vi "M100DailyOutputAuto.vi"() -> ()   [LabVIEW 2012]
uses:
  <vilib>/addons/database/Connection.llb/DB Tools Open Connec (Path).vi
  <vilib>/addons/database/Connection.llb/Conn Execute.vi
  <vilib>/addons/database/Recordset.llb/Rec Fetch Recordset Data (R).vi
  <vilib>/addons/database/Recordset.llb/Rec Destroy - Connection.vi
  <vilib>/Utility/file.llb/Write To Spreadsheet File (string).vi
  <vilib>/addons/database/_DB Variant To Data/Database Variant To Data.xnode
  <vilib>/addons/database/NI_Database_API.lvlib
  <vilib>/Utility/SMTP/NI_SMTPEmail.lvlib
panel:
  out "error out":errorcluster
  out "Array 2":string[][](array[string])
  out "spreadsheet string":string
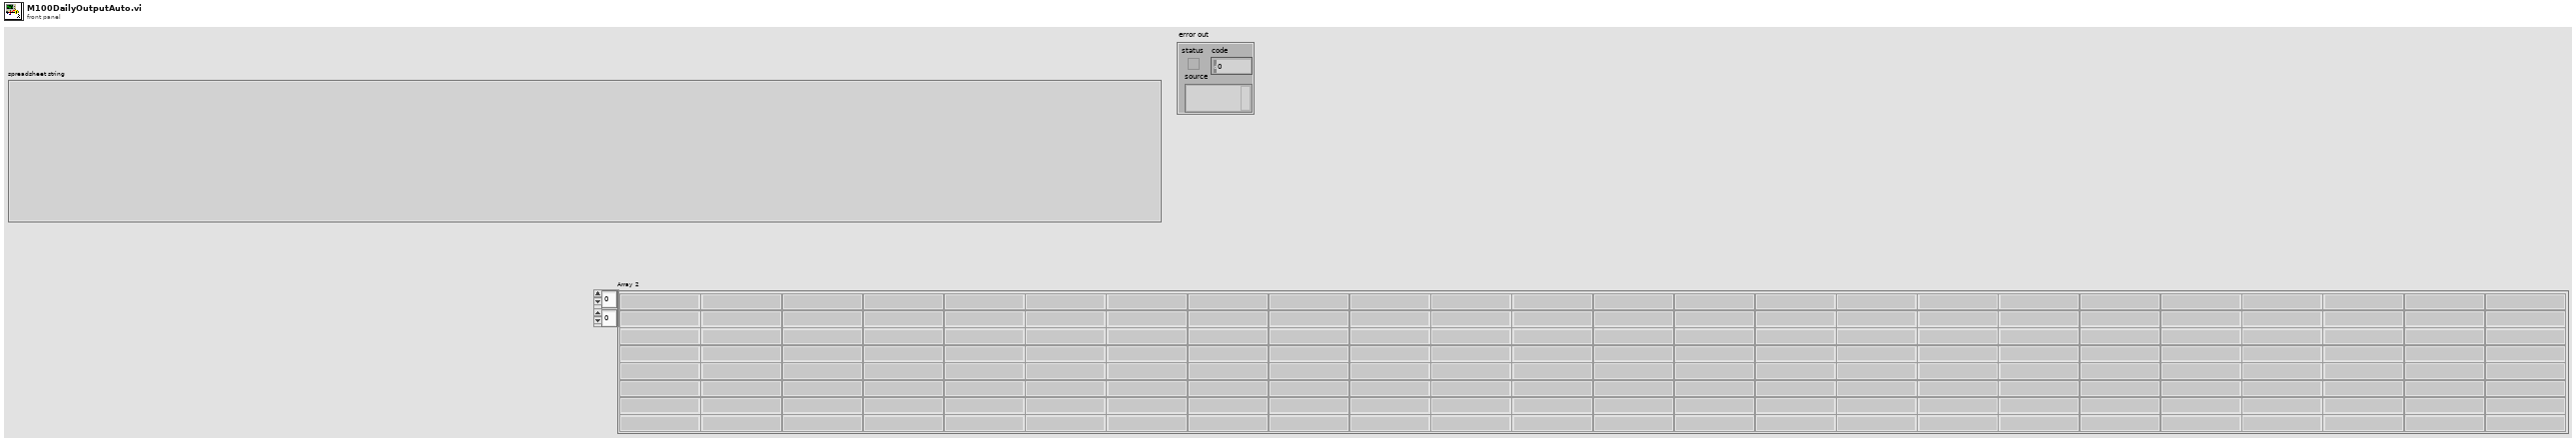
[diagram p1: front panel]
types:
  T1 = typedef "NI_Database_API.lvlib/Conn ObjectReference.ctl" = refnum<k1>
  T2 = typedef "NI_Database_API.lvlib/Rec ObjectReference.ctl" = refnum<k1>
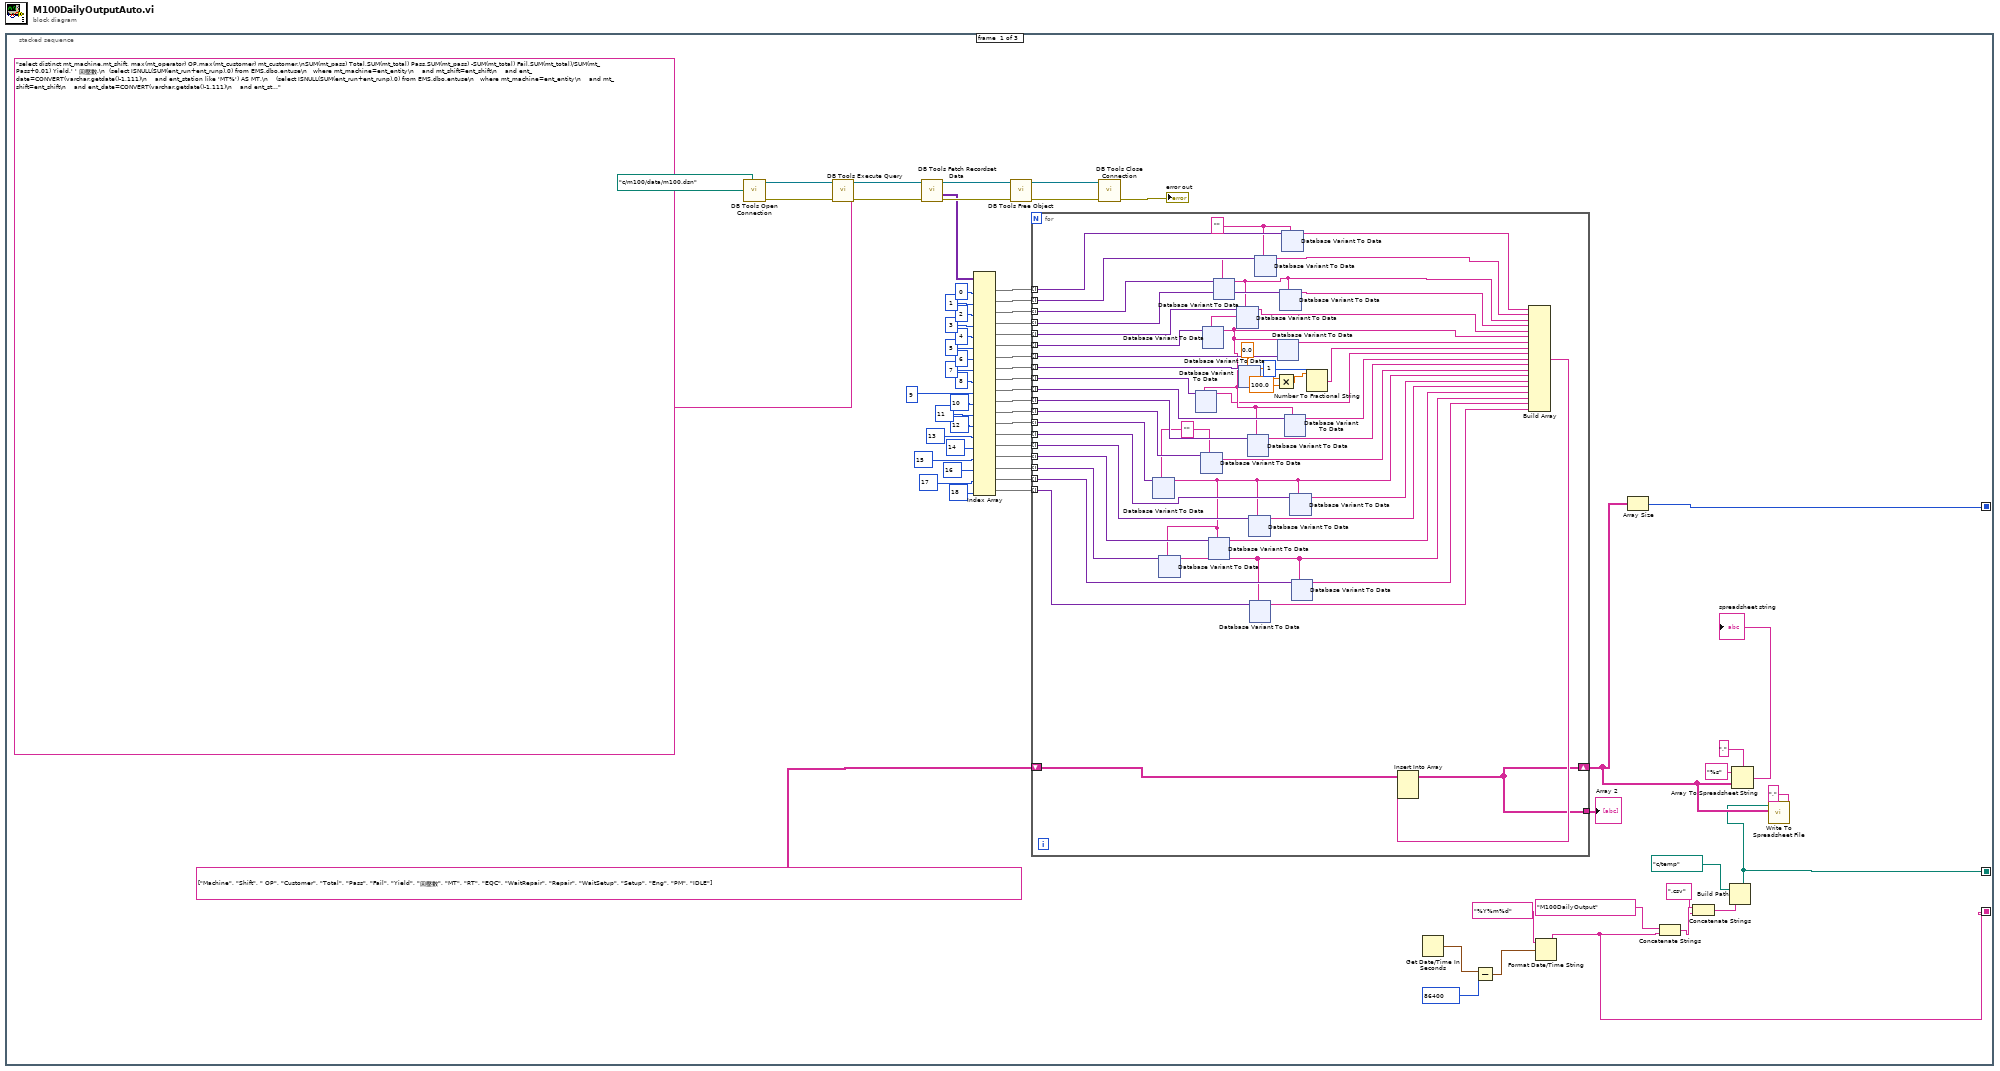
[diagram p0: block diagram]
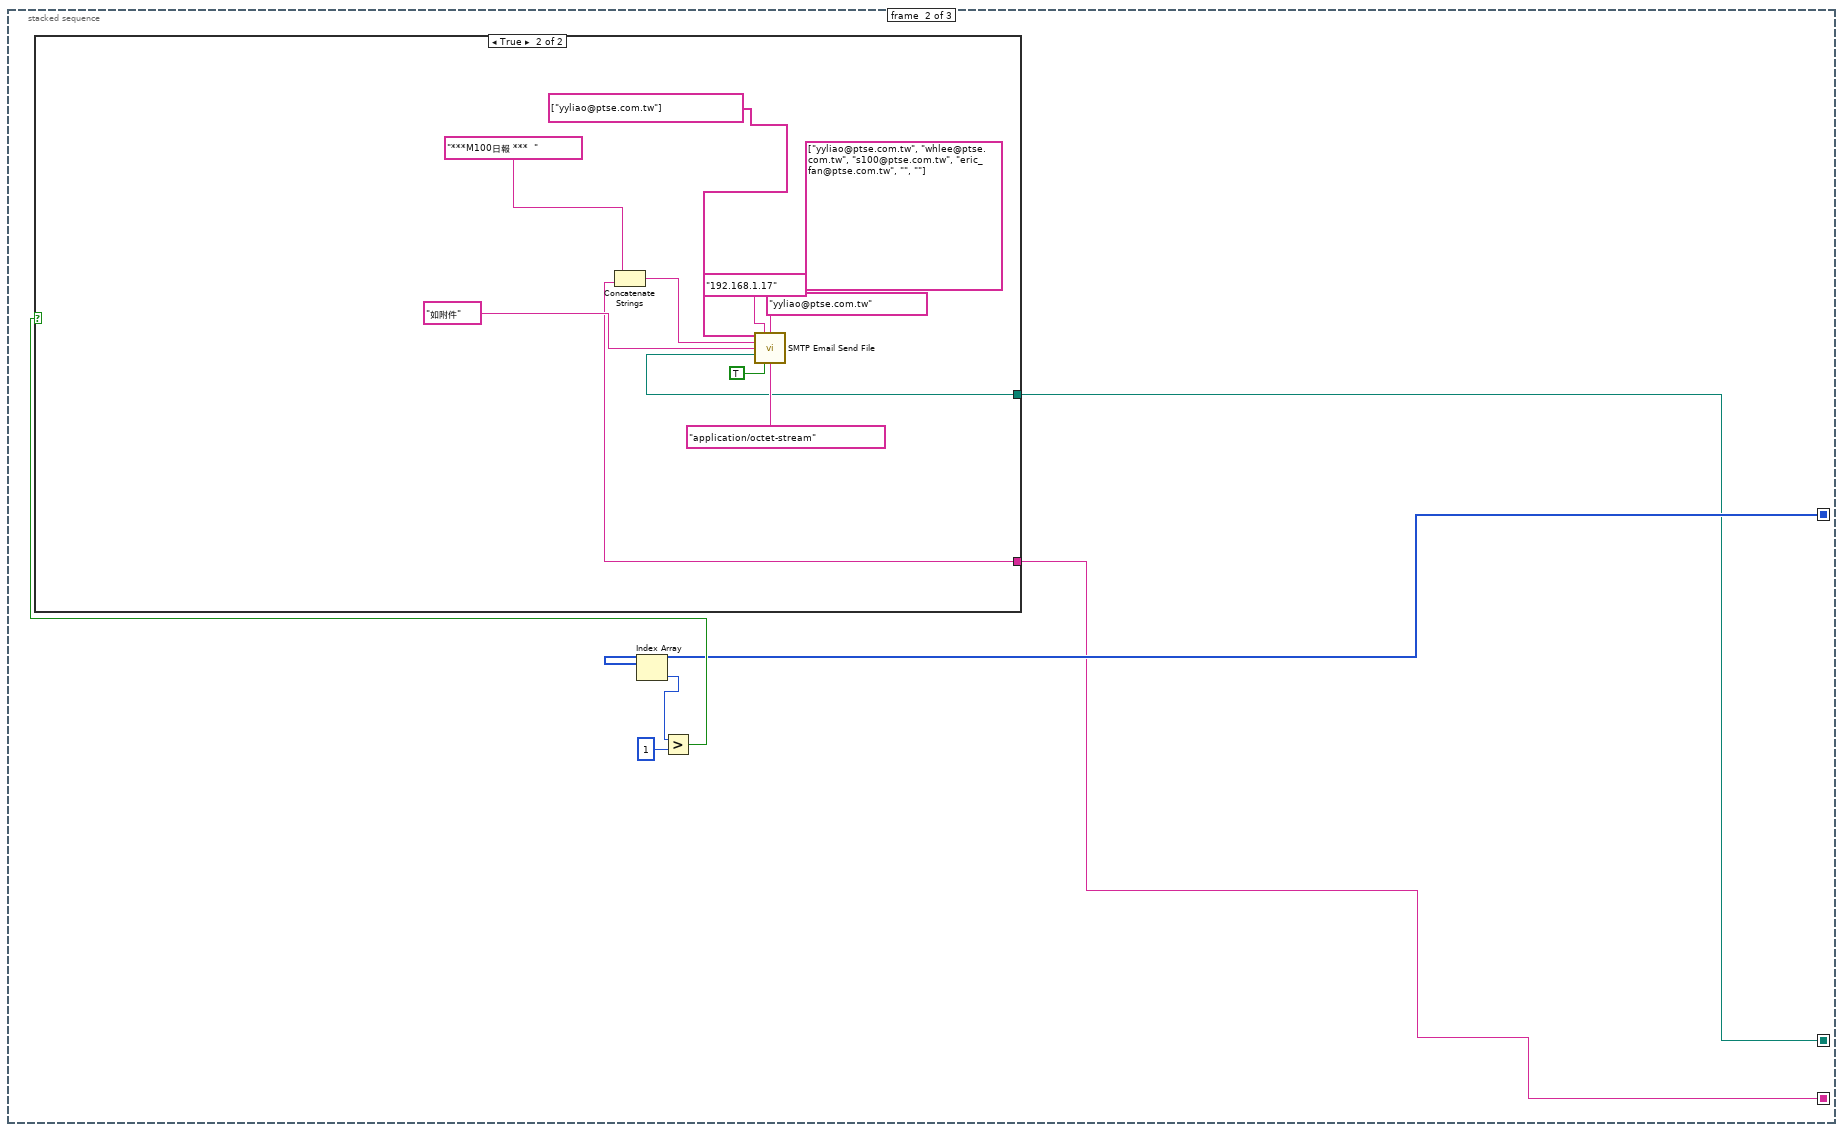
[diagram p2: hidden frame]
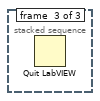
[diagram p4: hidden frame]
diagram:
  n1 = stacked-sequence {
    seq-local: [w37 _ _] -> [_ w728 _]
    seq-local: [w8 _ _] -> [_ w727 _]
    seq-local: [w4 _ _] -> [_ w726 _]
    frame #0 {
      n2 = call-poly <vilib>:"DB Tools Open Connection.vi"("connection information"=path "c:/m100/data/m100.dsn") -> ("error out"=w64:errorcluster, "connection reference"=w68:T1)  [unwired: 7 in]
      n3 = call-poly <vilib>:"DB Tools Execute Query.vi"("error in (no error)"=w64, "SQL query"="select distinct mt_machine,mt_shift, max(mt_operator) OP,max(mt_customer) mt_customer,\nSUM(mt_pass) Total,SUM(mt_total) Pass,SUM(mt_pass) -SUM(mt_total) Fail,SUM(mt_total)/SUM(mt_Pass+0.01) Yield,' ' 回壓數,\n  (select ISNULL(SUM(ent_run+ent_runp),0) from EMS.dbo.entuse\n   where mt_machine=ent_entity\n    and mt_shift=ent_shift\n    and ent_date=CONVERT(varchar,getdate()-1,111)\n    and ent_station like 'MT%') AS MT,\n    (select ISNULL(SUM(ent_run+ent_runp),0) from EMS.dbo.entuse\n   where mt_machine=ent_entity\n    and mt_shift=ent_shift\n    and ent_date=CONVERT(varchar,getdate()-1,111)\n    and ent_station like 'RT%') AS RT,\n    (select ISNULL(SUM(ent_run+ent_runp),0) from EMS.dbo.entuse\n   where mt_machine=ent_entity\n    and mt_shift=ent_shift\n    and ent_date=CONVERT(varchar,getdate()-1,111)\n    and ent_station like 'EQ%') AS EQC,\n    (select ISNULL(SUM(ent_wait_repair),0) from EMS.dbo.entuse\n   where mt_machine=ent_entity\n    and mt_shift=ent_shift\n    and ent_date=CONVERT(varchar,getdate()-1,111)) as WaitRepair,\n     (select ISNULL(SUM(ent_repair),0) from EMS.dbo.entuse\n   where mt_machine=ent_entity\n    and mt_shift=ent_shift\n    and ent_date=CONVERT(varchar,getdate()-1,111)) as Repair,\n    (select ISNULL(SUM(ent_wait_setup),0) from EMS.dbo.entuse\n   where mt_machine=ent_entity\n    and mt_shift=ent_shift\n    and ent_date=CONVERT(varchar,getdate()-1,111)) as WaitSetup,\n     (select ISNULL(SUM(ent_setup),0) from EMS.dbo.entuse\n   where mt_machine=ent_entity\n    and mt_shift=ent_shift\n    and ent_date=CONVERT(varchar,getdate()-1,111)) as Setup,\n    (select ISNULL(SUM(ent_eng),0) from EMS.dbo.entuse\n   where mt_machine=ent_entity\n    and mt_shift=ent_shift\n    and ent_date=CONVERT(varchar,getdate()-1,111)) as Eng,\n     (select ISNULL(SUM(ent_pm),0) from EMS.dbo.entuse\n   where mt_machine=ent_entity\n    and mt_shift=ent_shift\n    and ent_date=CONVERT(varchar,getdate()-1,111)) as PM,\n    (select ISNULL(SUM(ent_idle),0) from EMS.dbo.entuse\n   where mt_machine=ent_entity\n    and mt_shift=ent_shift\n    and ent_date=CONVERT(varchar,getdate()-1,111)) as IDLE\n  from m100.dbo.mt_data\n  where CONVERT(varchar,mt_end,111)=CONVERT(varchar,getdate()-1,111)\n    and mt_machine like 'QAMT%'\n  group by mt_machine,mt_shift\n  order by mt_machine,mt_shift desc", "connection reference"=w68) -> ("error out"=w63:errorcluster, "recordset reference"=w67:T2)  [unwired: 5 in]
      n4 = call-poly <vilib>:"DB Tools Fetch Recordset Data.vi"("error in (no error)"=w63, "recordset reference"=w67) -> ("error out"=w62:errorcluster, "recordset data"=w31:variant[][], "recordset reference out"=w66:T2)  [unwired: 3 in]
      n5 = Index Array(array=w31, index (col) #1=0 ("disabled index (col)"), index (col) #2=1 ("index (col)"), index (col) #3=2 ("index (col)"), index (col) #4=3 ("index (col)"), index (col) #5=4 ("index (col)"), index (col) #6=5 ("index (col)"), index (col) #7=6 ("index (col)"), index (col) #8=7 ("index (col)"), index (col) #9=8 ("index (col)"), index (col) #10=9 ("index (col)"), index (col) #11=10 ("index (col)"), index (col) #12=11 ("index (col)"), index (col) #13=12 ("index (col)"), index (col) #14=13 ("index (col)"), index (col) #15=14 ("index (col)"), index (col) #16=15 ("index (col)"), index (col) #17=16 ("index (col)"), index (col) #18=17 ("index (col)"), index (col) #19=18 ("index (col)")) -> (element #1=w48:variant[], element #2=w47:variant[], element #3=w46:variant[], element #4=w45:variant[], element #5=w44:variant[], element #6=w43:variant[], element #7=w42:variant[], element #8=w41:variant[], element #9=w40:variant[], element #10=w39:variant[], element #11=w38:variant[], element #12=w34:variant[], element #13=w33:variant[], element #14=w25:variant[], element #15=w24:variant[], element #16=w23:variant[], element #17=w22:variant[], element #18=w21:variant[], element #19=w1:variant[])  [unwired: 19 in]
      n6 = call-poly <vilib>:"DB Tools Free Object.vi"("error in (no error)"=w62, "recordset reference"=w66) -> ("error out"=w61:errorcluster, "connection reference"=w65:T1)  [unwired: 8 in]
      n7 = for {
        tunnel: w48 -> [w117] mode=indexing
        tunnel: w47 -> [w116] mode=indexing
        tunnel: w46 -> [w115] mode=indexing
        tunnel: w45 -> [w114] mode=indexing
        tunnel: w44 -> [w113] mode=indexing
        tunnel: w43 -> [w112] mode=indexing
        tunnel: w42 -> [w111] mode=indexing
        tunnel: w41 -> [w110] mode=indexing
        tunnel: w40 -> [w109] mode=indexing
        tunnel: w39 -> [w108] mode=indexing
        tunnel: w38 -> [w107] mode=indexing
        tunnel: [w104] -> w20
        shift-right: [w104] -> w16
        shift-left: string[][] [["Machine", "Shift", " OP", "Customer", "Total", "Pass", "Fail", "Yield", "回壓數", "MT", "RT", "EQC", "WaitRepair", "Repair", "WaitSetup", "Setup", "Eng", "PM", "IDLE"]] ("Array") -> [w103]
        tunnel: w34 -> [w102] mode=indexing
        tunnel: w33 -> [w101] mode=indexing
        tunnel: w25 -> [w88] mode=indexing
        tunnel: w24 -> [w87] mode=indexing
        tunnel: w23 -> [w86] mode=indexing
        tunnel: w22 -> [w85] mode=indexing
        tunnel: w21 -> [w84] mode=indexing
        tunnel: w1 -> [w78] mode=indexing
        w100 = ""
        w97 = ""
        n8 = xnode "Database Variant To Data"("database variant"=w101, "type"=w100) -> ("data"=w83:string)  [unwired: 1 in, 1 out]
        n9 = xnode "Database Variant To Data"("database variant"=w85, "type"=w83) -> ("data"=w77:string)  [unwired: 1 in, 1 out]
        n10 = xnode "Database Variant To Data"("database variant"=w102, "type"=w100) -> ("data"=w99:string)  [unwired: 1 in, 1 out]
        n11 = xnode "Database Variant To Data"("database variant"=w86, "type"=w83) -> ("data"=w80:string)  [unwired: 1 in, 1 out]
        n12 = xnode "Database Variant To Data"("database variant"=w115, "type"=w97) -> ("data"=w94:string)  [unwired: 1 in, 1 out]
        n13 = xnode "Database Variant To Data"("database variant"=w112, "type"=w94) -> ("data"=w93:string)  [unwired: 1 in, 1 out]
        n14 = xnode "Database Variant To Data"("database variant"=w109, "type"=w93) -> ("data"=w91:string)  [unwired: 1 in, 1 out]
        n15 = xnode "Database Variant To Data"("database variant"=w113, "type"=w94) -> ("data"=w95:string)  [unwired: 1 in, 1 out]
        n16 = xnode "Database Variant To Data"("database variant"=w110, "type"=0.0) -> ("data"=w74:dbl)  [unwired: 1 in, 1 out]
        n17 = xnode "Database Variant To Data"("database variant"=w107, "type"=w93) -> ("data"=w89:string)  [unwired: 1 in, 1 out]
        n18 = xnode "Database Variant To Data"("database variant"=w87, "type"=w83) -> ("data"=w81:string)  [unwired: 1 in, 1 out]
        n19 = xnode "Database Variant To Data"("database variant"=w78, "type"=w77) -> ("data"=w76:string)  [unwired: 1 in, 1 out]
        n20 = xnode "Database Variant To Data"("database variant"=w116, "type"=w97) -> ("data"=w98:string)  [unwired: 1 in, 1 out]
        n21 = Multiply(x=w74, y=100.0) -> (x*y=w72:dbl)
        n22 = xnode "Database Variant To Data"("database variant"=w111, "type"=w93) -> ("data"=w92:string)  [unwired: 1 in, 1 out]
        n23 = xnode "Database Variant To Data"("database variant"=w114, "type"=w94) -> ("data"=w96:string)  [unwired: 1 in, 1 out]
        n24 = xnode "Database Variant To Data"("database variant"=w117, "type"=w97) -> ("data"=w106:string)  [unwired: 1 in, 1 out]
        n25 = xnode "Database Variant To Data"("database variant"=w108, "type"=w93) -> ("data"=w90:string)  [unwired: 1 in, 1 out]
        n26 = xnode "Database Variant To Data"("database variant"=w88, "type"=w83) -> ("data"=w82:string)  [unwired: 1 in, 1 out]
        n27 = xnode "Database Variant To Data"("database variant"=w84, "type"=w77) -> ("data"=w79:string)  [unwired: 1 in, 1 out]
        n28 = Number To Fractional String(number=w72, precision (6)=i16 1) -> (F-format string=w70:string)  [unwired: 2 in]
        n29 = Build Array(w106, w98, w94, w96, w95, w93, w92, w70, w91, w90, w89, w99, w83, w82, w81, w80, w77, w79, w76) -> (w105:string[])
        n30 = Insert Into Array(array=w103, new element=w105) -> (w104:string[][])  [unwired: 2 in]
      }
      "Array 2" <- w20
      n31 = call <vilib>:"DB Tools Close Connection.vi"("error in (no error)"=w61, "connection reference"=w65) -> ("error out"=→"error out":errorcluster)  [unwired: 5 in]
      n32 = Get Date/Time In Seconds() -> (seconds since 1Jan1904=w7:timestamp)
      n33 = Subtract(x=w7, y=86400) -> (x-y=w5:timestamp)
      n34 = Format Date/Time String(time format string (%c)="%Y%m%d", seconds (now)=w5) -> (date/time string=w8:string)  [unwired: 1 in]
      n35 = Array Size(array=w16) -> (size(s)=w37:i32[])
      n36 = Concatenate Strings("M100DailyOutput" ("string"), w8) -> (w12:string)
      n37 = Concatenate Strings(w12, ".csv" ("string")) -> (w10:string)
      n38 = Build Path(base path=path "c:/temp", name or relative path=w10) -> (appended path=w4:path)
      n39 = Array To Spreadsheet String(delimiter (Tab)=",", array=w16, 3:"%s" ("format string")) -> (spreadsheet string=→"spreadsheet string":string)
      n40 = call-poly <vilib>:"Write To Spreadsheet File.vi"("delimiter (\\t)"="," ("delimiter (\\t)"), "2D data"=w16, "file path (dialog if empty)"=w4) -> ()  [unwired: 5 in, 1 out]
    }
    frame #1 {
      n41 = Index Array(array=w728) -> (element=w731:i32)  [unwired: 1 in]
      n42 = Greater?(x=w731, y=1) -> (0:w729:bool)
      n43 = case shown="True" w729 {
        tunnel: w726 -> [_ w736]
        tunnel: w727 -> [_ w732]
        frame False {
        }
        frame True {
          (unwired) string[] ["yyliao@ptse.com.tw", "whlee@ptse.com.tw", "s100@ptse.com.tw", "eric_fan@ptse.com.tw", "", ""] ("recipients")
          n44 = Concatenate Strings("***M100日報 ***  " ("subject ([No Subject])"), w732) -> (w734:string)
          n45 = call <vilib>:"SMTP Email Send File.vi"("recipients"=string[] ["yyliao@ptse.com.tw"], "mail server"="192.168.1.17", "return address"="yyliao@ptse.com.tw", "subject ([No Subject])"=w734, "message"="如附件", "file path"=w736, "binary? (F)"=TRUE, "MIME content-type (application/octet-stream)"="application/octet-stream") -> ()  [unwired: 6 in, 2 out]
        }
      }
    }
    frame #2 {
      n46 = Quit LabVIEW() -> ()  [unwired: 1 in]
    }
  }
